vi "refNewton Raphson Inner Part numeric derivative.vi"(4 "h":dbl=1e-08, 5 "NR Settings":cluster{"accuracy":dbl, "max iterations":i32}={"accuracy"=1e-08, "max iterations"=200}, 6 "end/start":dbl format="%.2f", 7 "level":dbl, 8 "case":bool, 9 "start/end":dbl format="%.2f", 10 "Variant":variant, 11 "function refnum":T1) -> (0 "error":i32, 1 "f(zero)":dbl format="%.2f", 2 "f'(zero)":dbl, 3 "zero":dbl format="%.2f")   [LabVIEW 2014, in "NI_Gmath.lvlib"]
uses:
  NI_Gmath.lvlib
  functionRefnum.ctl
panel:
  out "NaN/Path/Refnum?":bool
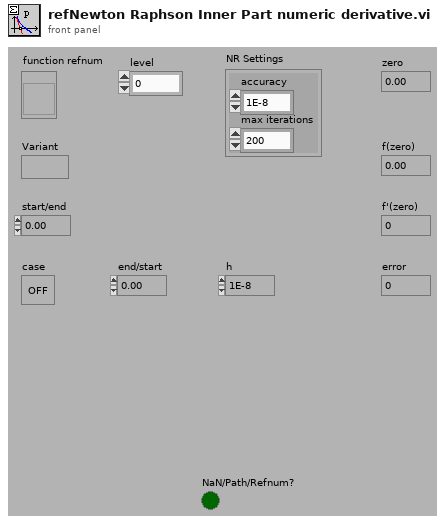
[diagram p1: front panel]
types:
  T1 = typedef "NI_Gmath.lvlib/functionRefnum.ctl" = refnum<vi>
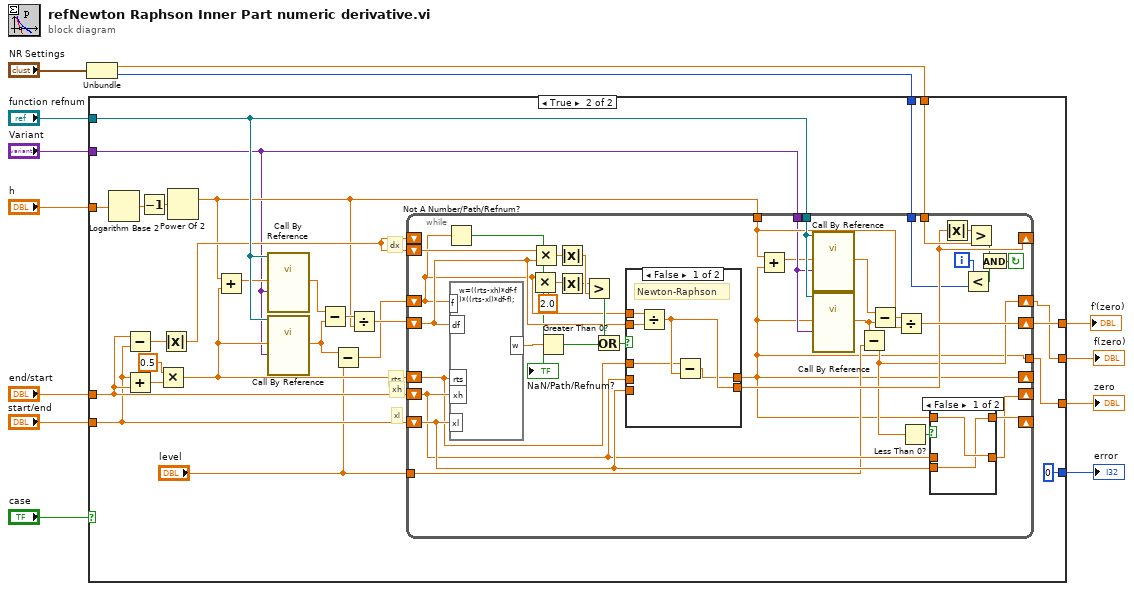
[diagram p0: block diagram]
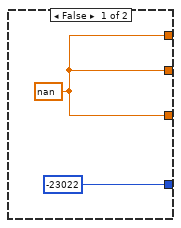
[diagram p2: hidden frame]
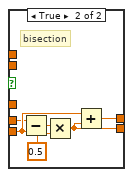
[diagram p4: hidden frame]
diagram:
  n1 = Unbundle("NR Settings") -> ("accuracy"=w2:dbl, "max iterations"=w1:i32)
  n2 = case shown="True" "case" {
    tunnel: [w14 w16] -> w8
    tunnel: [w14 w17] -> w7
    tunnel: "end/start" -> [_ w40]
    tunnel: "start/end" -> [_ w39]
    tunnel: "h" -> [_ w31]
    tunnel: w2 -> [_ w30]
    tunnel: [-23022 0] -> w11
    tunnel: "function refnum" -> [_ w41]
    tunnel: "Variant" -> [_ w23]
    tunnel: [w14 w26] -> w4
    tunnel: w1 -> [_ w21]
    frame False {
      w14 = nan
    }
    frame True {
      # "rts"
      # "dx"
      # "xh"
      # "xl"
      n3 = Logarithm Base 2(1:w31) -> (0:w34:dbl)
      n4 = Subtract(x=w40, y=w39) -> (x-y=w38:dbl)
      n5 = Add(x=w39, y=w40) -> (x+y=w28:dbl)
      n6 = Decrement(x=w34) -> (x-1=w33:dbl)
      n7 = Multiply(x=0.5, y=w28) -> (x*y=w25:dbl)
      n8 = Absolute Value(x=w38) -> (abs(x)=w37:dbl)
      n9 = Power Of 2(x=w33) -> (2^x=w32:dbl)
      n10 = Add(x=w32, y=w25) -> (x+y=w24:dbl)
      n11 = call-by-ref "?"(reference=w41, "Variant"=w23, "x"=w24) -> ("f(x)"=w22:dbl)  [unwired: 4 in, 2 out]
      n12 = call-by-ref "?"(reference=w41, "Variant"=w23, "x"=w25) -> ("f(x)"=w19:dbl)  [unwired: 4 in, 2 out]
      n13 = Subtract(x=w22, y=w19) -> (x-y=w36:dbl)
      n14 = Subtract(x=w19, y="level") -> (x-y=w20:dbl)
      n15 = Divide(x=w36, y=w32) -> (x/y=w35:dbl)
      n16 = while {
        tunnel: w32 -> [w60]
        tunnel: w30 -> [w64]
        shift-left: w37 -> [w63]
        shift-left: w39 -> [w69]
        shift-right: [w67] -> _
        shift-left: w40 -> [w68]
        shift-right: [w66] -> _
        shift-left: w35 -> [w71]
        shift-right: [w59] -> w26
        shift-left: w20 -> [w51]
        shift-right: [w44] -> w17
        shift-left: w37 -> [_]
        shift-right: [w57] -> _
        shift-left: w25 -> [w65]
        shift-right: [w42] -> _
        tunnel: w41 -> [w78]
        tunnel: w23 -> [w49]
        tunnel: w21 -> [w48]
        tunnel: "level" -> [w45]
        tunnel: [w42] -> w16
        i -> [w55]
        stop <- w52 continue-if-true
        n17 = Not A Number/Path/Refnum?(number/path/refnum=w51) -> (NaN/Path/Refnum?=→"NaN/Path/Refnum?":bool)
        n18 = formula code="w=((rts-xh)*df-f)*((rts-xl)*df-f);"("f"=w51, "df"=w71, "rts"=w65, "xh"=w68, "xl"=w69) -> ("w"=w56:dbl)
        n19 = Multiply(x=w51, y=2.0) -> (x*y=w75:dbl)
        n20 = Multiply(x=w63, y=w71) -> (x*y=w76:dbl)
        n21 = Greater Than 0?(x=w56) -> (x > 0?=w58:bool)
        n22 = Absolute Value(x=w76) -> (abs(x)=w79:dbl)
        n23 = Absolute Value(x=w75) -> (abs(x)=w74:dbl)
        n24 = Greater?(x=w74, y=w79) -> (0:w73:bool)
        n25 = Or(x=w73, y=w58) -> (x .or. y?=w72:bool)
        n26 = case shown="False" w72 {
          tunnel: w68 -> [_ w93]
          tunnel: w69 -> [_ w94]
          tunnel: [w88 w90] -> w57
          tunnel: [w84 w89] -> w42
          tunnel: w51 -> [w87 _]
          tunnel: w71 -> [w86 _]
          tunnel: w65 -> [w85 _]
          frame False {
            # "Newton-Raphson"
            n27 = Divide(x=w87, y=w86) -> (x/y=w88:dbl)
            n28 = Subtract(x=w85, y=w88) -> (x-y=w84:dbl)
          }
          frame True {
            # "bisection"
            n29 = Subtract(x=w93, y=w94) -> (x-y=w92:dbl)
            n30 = Multiply(x=w92, y=0.5) -> (x*y=w90:dbl)
            n31 = Add(x=w94, y=w90) -> (x+y=w89:dbl)
          }
        }
        n32 = Add(x=w60, y=w42) -> (x+y=w43:dbl)
        n33 = call-by-ref "?"(reference=w78, "Variant"=w49, "x"=w43) -> ("f(x)"=w47:dbl)  [unwired: 4 in, 2 out]
        n34 = call-by-ref "?"(reference=w78, "Variant"=w49, "x"=w42) -> ("f(x)"=w46:dbl)  [unwired: 4 in, 2 out]
        n35 = Subtract(x=w46, y=w45) -> (x-y=w44:dbl)
        n36 = Subtract(x=w47, y=w46) -> (x-y=w61:dbl)
        n37 = Divide(x=w61, y=w60) -> (x/y=w59:dbl)
        n38 = Less Than 0?(x=w44) -> (x < 0?=w70:bool)
        n39 = case shown="False" w70 {
          tunnel: w69 -> [w80 _]
          tunnel: w68 -> [_ w82]
          tunnel: w42 -> [w81 w83]
          tunnel: [w80 w83] -> w67
          tunnel: [w81 w82] -> w66
          frame False {
          }
          frame True {
          }
        }
        n40 = Absolute Value(x=w57) -> (abs(x)=w62:dbl)
        n41 = Less?(x=w55, y=w48) -> (x < y?=w54:bool)
        n42 = Greater?(x=w62, y=w64) -> (0:w53:bool)
        n43 = And(x=w53, y=w54) -> (x .and. y?=w52:bool)
      }
    }
  }
  "error" <- w11
  "zero" <- w8
  "f(zero)" <- w7
  "f'(zero)" <- w4
